vi "VideoCapture CopyLastFrame.vi"(4 "Image Type":T1, 6 "height":i32, 8 "error in (no error)":errorcluster, 9 "width":i32, 10 "Image":T2, 11 "VideoCapture in":refnum<class "VideoCapture.lvclass">) -> (0 "error out":errorcluster, 2 "Image":T2, 3 "VideoCapture out":refnum<class "VideoCapture.lvclass">)   [LabVIEW 2020, in "OpenLvVision_OpenCv.lvlib" / "VideoCapture.lvclass"]
uses:
  VideoCapture.lvclass
  C:/Users/lukas/Downloads/OpenLvVision_OpenCv/SourceCode/LabView/OpenLvVision_OpenCv/_LvHelpers/EdvrObject/EdvrObject.lvclass
  <vilib>/vision/Image Controls.llb/IMAQ Image.ctl
  <vilib>/OpenLvVision/OpenLvVision_Image/Management/TypeDef/OLV ImageType.ctl
  _LvHelpers/EdvrObject/EdvrObject.lvclass/EdvrObject.ctl
  _LvHelpers/MatHandling/RegisterMat/RegisterMat_Image.vi
  _LvHelpers/MatHandling/UnregisterMat/UnregisterMat_Image.vi
  _LvHelpers/EdvrObject/EdvrObject.lvclass
  Dlls/OlvOpenCvWrapper.dll
  OpenLvVision_OpenCv.lvlib
  <vilib>/OpenLvVision/OpenLvVision_Image/Management/OLV Management.lvlib
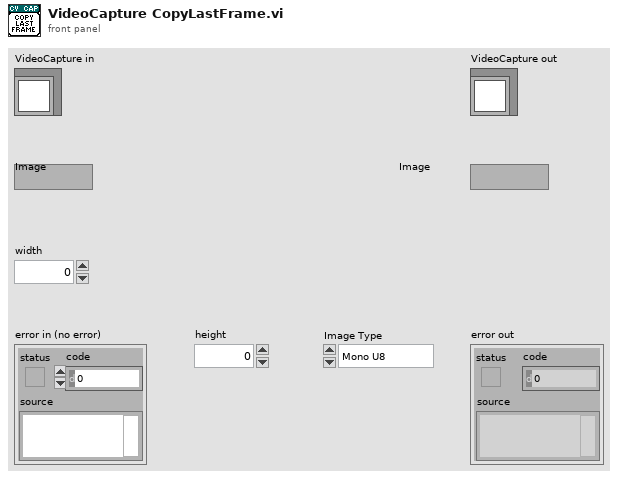
[diagram p1: front panel]
types:
  T1 = typedef "OLV OpenLvVision_Image.lvlib/OLV Management.lvlib/OLV ImageType.ctl" = enum16{"Mono U8", "Mono U16", "Mono I16", "Mono SGL", "Color U32", "Color U64", "Complex CSG"}
  T2 = typedef "IMAQ Image.ctl" = refnum<image>
  T3 = typedef "OLV OpenLvVision_Image.lvlib/OLV Management.lvlib/OLV Image.ctl" = refnum<image>
  T4 = typedef "OpenLvVision_OpenCv.lvlib/MatInfo.ctl" = cluster{"Datatype":T5, "Height":i32, "Width":i32, "Channels":i32, "LineWidth":i32, "Null":u8}
  T5 = typedef "OpenLvVision_OpenCv.lvlib/LvDatatype.ctl" = enum32{"Undefined", "U8", "I8", "U16", "I16", "U32_Color", "I32", "U64_Color", "I64", "SGL", "DBL", "Complex SGL", "Complex DBL", "Array 1D U8", "Array 1D I8", "Array 1D U16", "Array 1D I16", "Array 1D U32_Color", "Array 1D I32", "Array 1D U64_Color", "Array 1D I64", "Array 1D SGL", "Array 1D DBL", "Array 1D Complex SGL", "Array 1D Complex DBL", "Array 2D U8", "Array 2D I8", "Array 2D U16", "Array 2D I16", "Array 2D U32", "Array 2D U32_Color", "Array 2D I32", "Array 2D U64", "Array 2D U64_Color", "Array 2D I64", "Array 2D SGL", "Array 2D DBL", "Array 2D Complex SGL", "Array 2D Complex DBL", "Image Mono U8", "Image Mono U16", "Image Mono I16", "Image Mono SGL", "Image Color U32", "Image Color U64", "ImageComplex Sgl", "Array1d_2dPointI32", "Array1d_2dPointSGL", "Array1d_2dPointDBL", "Array1d_3dPointI32", "Array1d_3dPointSGL", "Array1d_3dPointDBL", "Array1d_4dPointI32", "Array1d_4dPointSGL", "Array1d_4dPointDBL", "ArrayNchwU8", "ArrayNchwI8", "ArrayNchwU16", "ArrayNchwI16", "ArrayNchwU32_Color", "ArrayNchwI32", "ArrayNchwU64_Color", "ArrayNchwSgl", "ArrayNchwDbl", "ArrayNchwComplexSgl", "ArrayNchwComplexDbl"}
  T6 = typedef "OpenLvVision_OpenCv.lvlib/EdvrObject.lvclass/Edvr.ctl" = refnum<data-value>
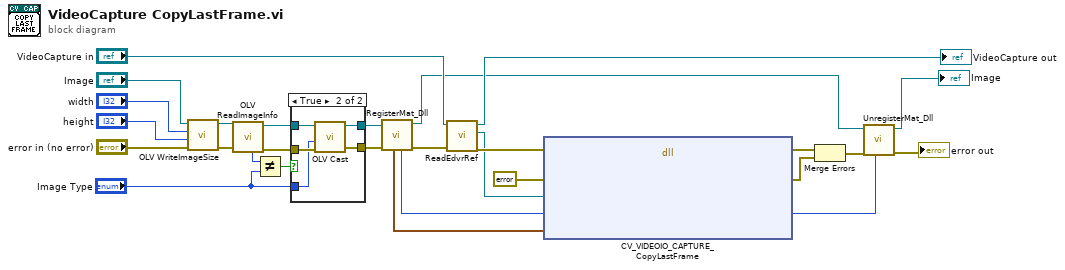
[diagram p0: block diagram]
diagram:
  n1 = call <vilib>:"OLV WriteImageSize.vi"("error in"="error in (no error)", "Height"="height", "Width"="width", "Image Reference In"="Image") -> ("error out"=w9:errorcluster, "Image Reference Out"=w5:T3)  [unwired: 6 in]
  n2 = call <vilib>:"OLV ReadImageInfo.vi"("error in"=w9, "Image Reference In"=w5) -> ("error out"=w11:errorcluster, "Image Reference Out"=w4:T3, "Image Type"=w2:T1)  [unwired: 4 in, 3 out]
  n3 = Not Equal?(x=w2, y="Image Type") -> (x != y?=w3:bool)
  n4 = case shown="True" w3 {
    tunnel: [w29 w35] -> w13
    tunnel: [w30 w34] -> w12
    tunnel: w11 -> [w29 w33]
    tunnel: w4 -> [w30 w32]
    tunnel: "Image Type" -> [_ w31]
    frame False {
    }
    frame True {
      n5 = call <vilib>:"OLV Cast.vi"("error in"=w33, "Image Type"=w31, "Image Src Reference In"=w32) -> ("error out"=w35:errorcluster, "Image Dst Reference Out"=w34:T3)  [unwired: 7 in]
    }
  }
  n6 = call-poly "RegisterMat_Dll.vi"("error in"=w13, "Image Reference In"=w12) -> ("error out"=w21:errorcluster, "Image Reference Out"=w18:T3, "AdressOrData"=w17:u64, "Mat"=w16:T4)  [unwired: 6 in]
  n7 = call "ReadEdvrRef.vi"("error in (no error)"=w21, "EdvrObject in"="VideoCapture in") -> ("error out"=w27:errorcluster, "Edvr"=w26:T6, "EdvrObject out"=→"VideoCapture out":refnum<class "VideoCapture.lvclass">)  [unwired: 7 in]
  n8 = dll-call lib="C:/Users/lukas/Downloads/OpenLvVision_OpenCv/SourceCode/LabView/OpenLvVision_OpenCv/Dlls/OlvOpenCvWrapper.dll" fn="CV_VIDEOIO_CAPTURE_CopyLastFrame"(error in=w27, "Error"=errorcluster {"status"=FALSE, "code"=0, "source"=""} ("error out"), "edvrRef"=w26, "addressDst"=w17, "matInfoDst"=w16) -> (error out=w23:errorcluster, "Error"=w22:errorcluster, "addressDst"=w15:u64)  [unwired: 5 in, 1 out]
  n9 = Merge Errors(w23, w22) -> (w20:errorcluster)
  n10 = call-poly "UnregisterMat_Dll.vi"("AdressOrData"=w15, "error in"=w20, "Image Reference In"=w18) -> ("error out"=→"error out":errorcluster, "Image Reference Out"=→"Image":T3)  [unwired: 7 in]
